vi "Delay_Global.vi"() -> ()   [LabVIEW 2021]
panel:
  in  "delay (default)":u32=10
  in  "extended delay":u32=500
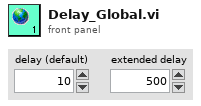
[diagram p1: front panel]
diagram:
